vi "Configure Main Page.vi"(0 "VISA resource name":refnum<visa-resource-name>, 1 "Unit Address (1)":i16=1, 5 "Parameters":u16[](array[ring])=[15, 16, 2, 4, 5, 22, 23, 24, 21, 14, 12, 13, 6, 7, 11, 10] items=["None", "Input 1 Value", "Input 2 Value", "Input 3 Value", "Set Point 1", "Set Point 2", "% Power 1", "% Power 2", "Tune Status 1", "Tune Status 2", "Time", "Date", "Digital Inputs", "Digital Outputs", "Time Remaining", "Current File", "Current Step", "Active Ch1 PID Set", "Active Ch2 PID Set", "Last Jump Step", "Jump Count", "WaitFor Status", "Step Type", "Target SP1", "Target SP2", "Inner Set Point", "Custom Message 1", "Custom Message 2", "Custom Message 3", "Custom Message 4", "Input 1 Cal. Offset", "Input 2 Cal. Offset", "Input 3 Cal. Offset"], 11 "error in (no error)":errorcluster {"code" format="%.0x"}) -> (4 "VISA resource name out":refnum<visa-resource-name>, 15 "error out":errorcluster {"code" format="%.0x"})   [LabVIEW 2010]
doc: "This VI configures parameters to appear on Main Page."
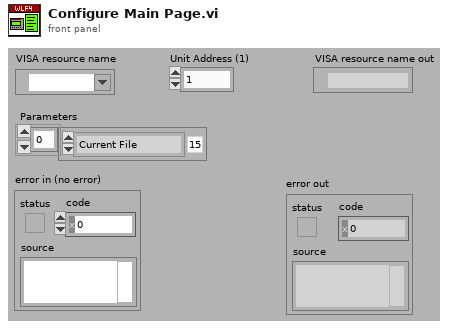
[diagram p1: front panel]
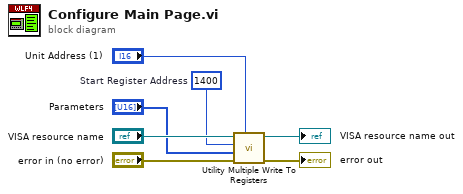
[diagram p0: block diagram]
diagram:
  w1 = u16 1400  # Start Register Address
  n1 = call "Utility Multiple Write To Registers.vi"("Unit Address (1)"="Unit Address (1)", "error in (no error)"="error in (no error)", "Array Of Data"="Parameters", "Register Address (0)"=w1, "VISA resource name"="VISA resource name") -> ("error out"=→"error out":errorcluster, "VISA resource name out"=→"VISA resource name out":refnum<visa-resource-name>)  [unwired: 5 in]
